vi "subHamamatsu_TurnOnOff.vi"(5 "logic 2":bool, 7 "logic 1":bool, 8 "error in (no error)":errorcluster, 11 "Handle in":u32) -> (0 "error out":errorcluster, 2 "Buffer":T1, 3 "Handle out":u32)   [LabVIEW 2015]
panel:
  # "logic1   logic2     Cam action         \n    1           1         start capture\n    1           0         stop capture\n   0           1           do nothing\n   0           0           do nothing"
  # "On = True\nOff = False"
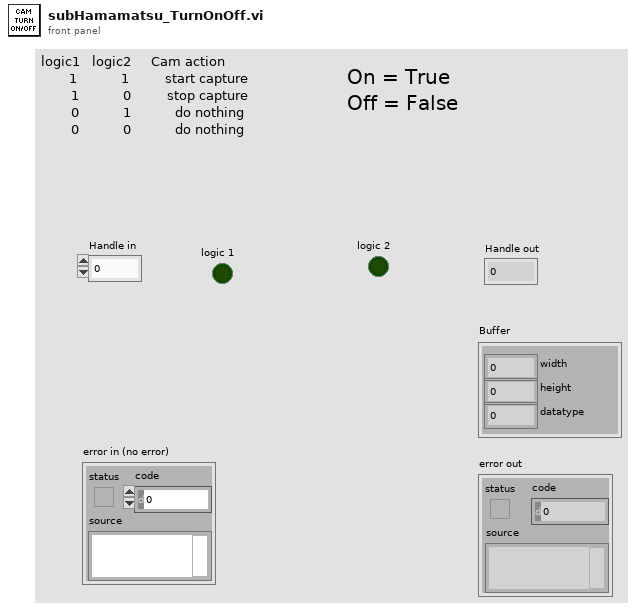
[diagram p1: front panel]
types:
  T1 = cluster{"width":u32, "height":u32, "datatype":u32}
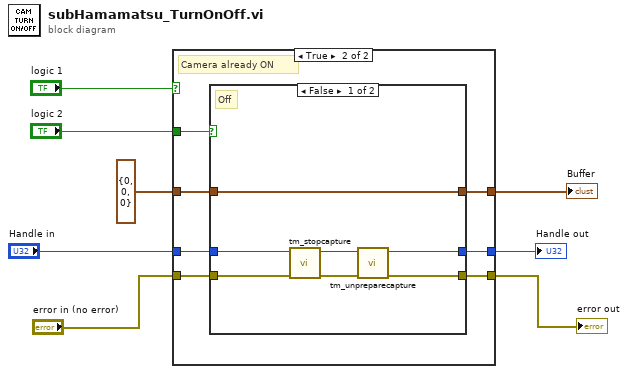
[diagram p0: block diagram]
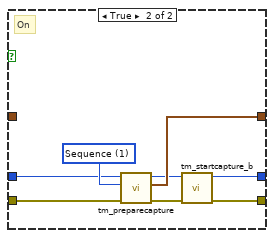
[diagram p3: hidden frame]
diagram:
  n1 = case shown="True" "logic 1" {
    tunnel: "Handle in" -> [w10 w12]
    tunnel: "error in (no error)" -> [w11 w18]
    tunnel: [w11 w17] -> w7
    tunnel: [w10 w16] -> w1
    tunnel: [w9 w15] -> w6
    tunnel: "logic 2" -> [_ w14]
    tunnel: T1 {"width"=0, "height"=0, "datatype"=0} ("Buffer") -> [w9 w13]
    frame False {
      # "Camera already OFF"
    }
    frame True {
      # "Camera already ON"
      n2 = case shown="False" w14 {
        tunnel: [w25 w31] -> w17
        tunnel: w18 -> [w24 w33]
        tunnel: w12 -> [w19 w26]
        tunnel: [w23 w32] -> w16
        tunnel: [w20 w30] -> w15
        tunnel: w13 -> [w20 _]
        frame False {
          # "Off"
          n3 = call "tm_stopcapture.vi"("error in (no error)"=w24, "Handle in"=w19) -> ("error out"=w21:errorcluster, "Handle out"=w22:u32)  [unwired: 8 in]
          n4 = call "tm_unpreparecapture.vi"("error in (no error)"=w21, "Handle in"=w22) -> ("error out"=w25:errorcluster, "Handle out"=w23:u32)  [unwired: 8 in]
        }
        frame True {
          w27 = 1 items=["Snap", "Sequence"] ("Capture mode")
          # "On"
          n5 = call "tm_preparecapture.vi"("error in (no error)"=w33, "Capture mode"=w27, "Handle in"=w26) -> ("error out"=w29:errorcluster, "Buffer"=w30:T1, "Handle out"=w28:u32)  [unwired: 5 in, 1 out]
          n6 = call "tm_startcapture_b.vi"("error in (no error)"=w29, "Handle in"=w28) -> ("error out"=w31:errorcluster, "Handle out"=w32:u32)  [unwired: 8 in]
        }
      }
    }
  }
  "error out" <- w7
  "Buffer" <- w6
  "Handle out" <- w1
